vi "Teleop.vi"(10 "Match Info":T1={"Autonomous Elapsed Seconds"=0.0, "TeleOp Elapsed Seconds"=0.0, "Disabled Elapsed Seconds"=0.0, "Visited Autonomous"=FALSE, "Visited TeleOp"=FALSE, "Visited Disabled"=FALSE, "Autonomous Settings"={"Autonomous Style"=enum."Independent", "VI Refnum"=refnum}}, 11 "Call Context":T2) -> ()   [LabVIEW 2020]
doc: "This VI is called for each enabled TeleOp packet received from the DS. It is typically used to read from joysticks and other inputs and update I/O or setpoints for timed control loops. It should complete and return within 20 milliseconds or risk missing DS packets."
uses:
  <vilib>/Rock Robotics/WPI/DriverStation/WPI_DriverStationDerivedRobotMode.ctl
  <vilib>/Rock Robotics/WPI/DriverStation/WPI_DriverStationMatch Info.ctl
  Swerve/Implementation/Swerve Setpoints.ctl
  Swerve/Implementation/Swerve Operations.ctl
  Intake/Implementation/Intake Setpoints.ctl
  Intake/Implementation/Intake Operations.ctl
  <vilib>/Rock Robotics/WPI/Joystick/XBox Buttons Indexer.ctl
  <vilib>/Rock Robotics/WPI/Joystick/XBox Axes Indexer.ctl
  Climber/Implementation/Climber Operations.ctl
  Climber/Implementation/Climber Setpoints.ctl
  Shooter/Implementation/Shooter Operations.ctl
  Shooter/Implementation/Shooter Setpoints.ctl
  <vilib>/Rock Robotics/WPI/Utilities/WPI_GetSetVariantRefNum.vi
  <vilib>/Rock Robotics/Network Tables/NT Write Boolean Array.vi
  <vilib>/Rock Robotics/Network Tables/NT Write Numeric Array.vi
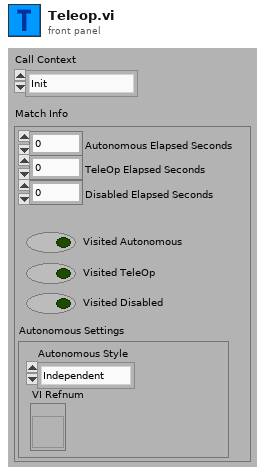
[diagram p1: front panel]
types:
  T1 = typedef "WPI_DriverStationMatch Info.ctl" = cluster{"Autonomous Elapsed Seconds":dbl, "TeleOp Elapsed Seconds":dbl, "Disabled Elapsed Seconds":dbl, "Visited Autonomous":bool, "Visited TeleOp":bool, "Visited Disabled":bool, "Autonomous Settings":cluster{"Autonomous Style":enum16{"Iterative", "Independent"}, "VI Refnum":refnum<vi>}}
  T2 = typedef "WPI_DriverStationDerivedRobotMode.ctl" = enum16{"Init", "Execute", "Stop"}
  T3 = typedef "XBox Buttons Indexer.ctl" = enum16{"A", "B", "X", "Y", "Left Bumper", "Right Bumper", "Back", "Start", "Left Joystick", "Right Joystick"}
  T4 = typedef "XBox Axes Indexer.ctl" = enum16{"Left X", "Left Y", "Left Trigger", "Right Trigger", "Right X", "Right Y"}
  T5 = typedef "Intake Setpoints.ctl" = cluster{"Operation":T6, "Numeric":dbl}
  T6 = typedef "Intake Operations.ctl" = enum16{"Reserve", "Read Current", "Immediate", "Retract", "Extend", "Feed"}
  T7 = typedef "Swerve Setpoints.ctl" = cluster{"Operation":T8, "Gyro":dbl, "X Rotate":dbl, "FWD":dbl, "STR":dbl, "Time":dbl, "Angle":dbl, "Distance":dbl, "Right Trigger":dbl, "Y Rotate":dbl, "Start Angle":dbl}
  T8 = typedef "Swerve Operations.ctl" = enum16{"Reserve", "Read Current", "Immediate", "Direct  Joystick Drive", "Joystick Drive", "Drive for Distance", "Drive for Time", "Turn to Angle", "Drive to Angle(Time)", "Drive to Angle(Distance)"}
  T9 = typedef "WPI_JoystickDevRef.ctl" = cluster{"Device":T10}
  T10 = typedef "WPI_JoystickDeviceEnum.ctl" = enum16{"USB 0", "USB 1", "USB 2", "USB 3", "USB 4", "USB 5"}
  T11 = typedef "Climber Setpoints.ctl" = cluster{"Operation":T12, "Numeric":dbl}
  T12 = typedef "Climber Operations.ctl" = enum16{"Reserve", "Read Current", "Immediate", "Unlock Winch", "Lock Winch", "Stop Winch", "Spool Winch", "Unspool Winch", "Arm Out", "Arm In", "Open Hook", "Close Hook"}
  T13 = typedef "ADIS16470 Device Reference.ctl" = cluster{"DevStatus":errorcluster, "Hardware Config":T14, "Calibration Complete":refnum<notifier>, "Status Reference":refnum<data-value>, "Data Reference":refnum<data-value>, "Sychronous Process VI":T18, "Cmd FIFO":refnum<k33>, "Source":T19, "Data FIFO":refnum<k33>, "Calibration Time (ms)":u32, "Data Reference":refnum<data-value>}
  T14 = typedef "ADIS16470 Hardware Configuration.ctl" = cluster{"SPI Clock Rate (Hz)":dbl, "IMU SPI Mode (3)":T15, "IMU Reset Pin":T16, "IMU SPI Bus":T17, "IMU Data Ready Pin":T16, "Stall Config":cluster{"Pow2BytesPerRead":u8, "StallTicks":u16, "CsToSclkTicks":u8}}
  T15 = typedef "WPI_SPIMode.ctl" = enum16{"Mode 0 (Clk Idle Low,Sample on Leading)", "Mode 1 (Clk Idle Low,Sample on Trailing)", "Mode 2 (Clk Idle High,Sample on Leading)", "Mode 3 (Clk Idle High,Sample on Trailing)"}
  T16 = typedef "FPGA_DIOChannel.ctl" = enum8{"DIO 0", "DIO 1", "DIO 2", "DIO 3", "DIO 4", "DIO 5", "DIO 6", "DIO 7", "DIO 8", "DIO 9", "DIO MXP 0", "DIO MXP 1", "DIO MXP 2", "DIO MXP 3", "DIO MXP 4", "DIO MXP 5", "DIO MXP 6", "DIO MXP 7", "DIO MXP 8", "DIO MXP 9", "DIO MXP 10", "DIO MXP 11", "DIO MXP 12", "DIO MXP 13", "DIO MXP 14", "DIO MXP 15", "SPI Port CS1", "SPI Port CS2", "SPI Port CS3", "SPI Port MISO", "SPI Port MOSI", "Invalid"}
  T17 = typedef "spi_bus.ctl" = enum16{"SPI On-Board, CS0", "SPI On-Board, CS1", "SPI On-Board, CS2", "SPI On-Board, CS3", "SPI MXP", "Invalid"}
  T18 = typedef "ADIS16470 Process.ctl" = refnum<vi>
  T19 = typedef "FPGA_CounterEncoderSourceConvertionLVSourceType.ctl" = cluster{"DevStatus":errorcluster, "AnalogTriggerMode?":bool, "DigitalMode":cluster{"DIO Channel":T20}, "AnalogTriggerMode":cluster{"AnalogTriggerIndex":T21, "OutputType":T22}}
  T20 = typedef "FPGA_DIODigitalSourceChannel.ctl" = enum8{"DIO 0", "DIO 1", "DIO 2", "DIO 3", "DIO 4", "DIO 5", "DIO 6", "DIO 7", "DIO 8", "DIO 9", "DIO MXP 0", "DIO MXP 1", "DIO MXP 2", "DIO MXP 3", "DIO MXP 4", "DIO MXP 5", "DIO MXP 6", "DIO MXP 7", "DIO MXP 8", "DIO MXP 9", "DIO MXP 10", "DIO MXP 11", "DIO MXP 12", "DIO MXP 13", "DIO MXP 14", "DIO MXP 15", "SPI Port CS1", "SPI Port CS2", "SPI Port CS3", "SPI Port MISO", "SPI Port MOSI", "Disabled"}
  T21 = typedef "FPGA_AnalogTriggerIndex.ctl" = enum8{"Trig 0", "Trig 1", "Trig 2", "Trig 3", "Trig 4", "Trig 5", "Trig 6", "Trig 7", "Invalid"}
  T22 = typedef "FPGA_AnalogTriggerOutType.ctl" = enum16{"InWindow", "TriggerState", "Rising", "Falling"}
  T23 = typedef "ADIS16470 Data.ctl" = cluster{"XAngle":dbl, "YAngle":dbl, "ZAngle":dbl}
  T24 = typedef "Shooter Setpoints.ctl" = cluster{"Operation":T25, "Numeric":dbl}
  T25 = typedef "Shooter Operations.ctl" = enum16{"Reserve", "Read Current", "Immediate", "Shoot"}
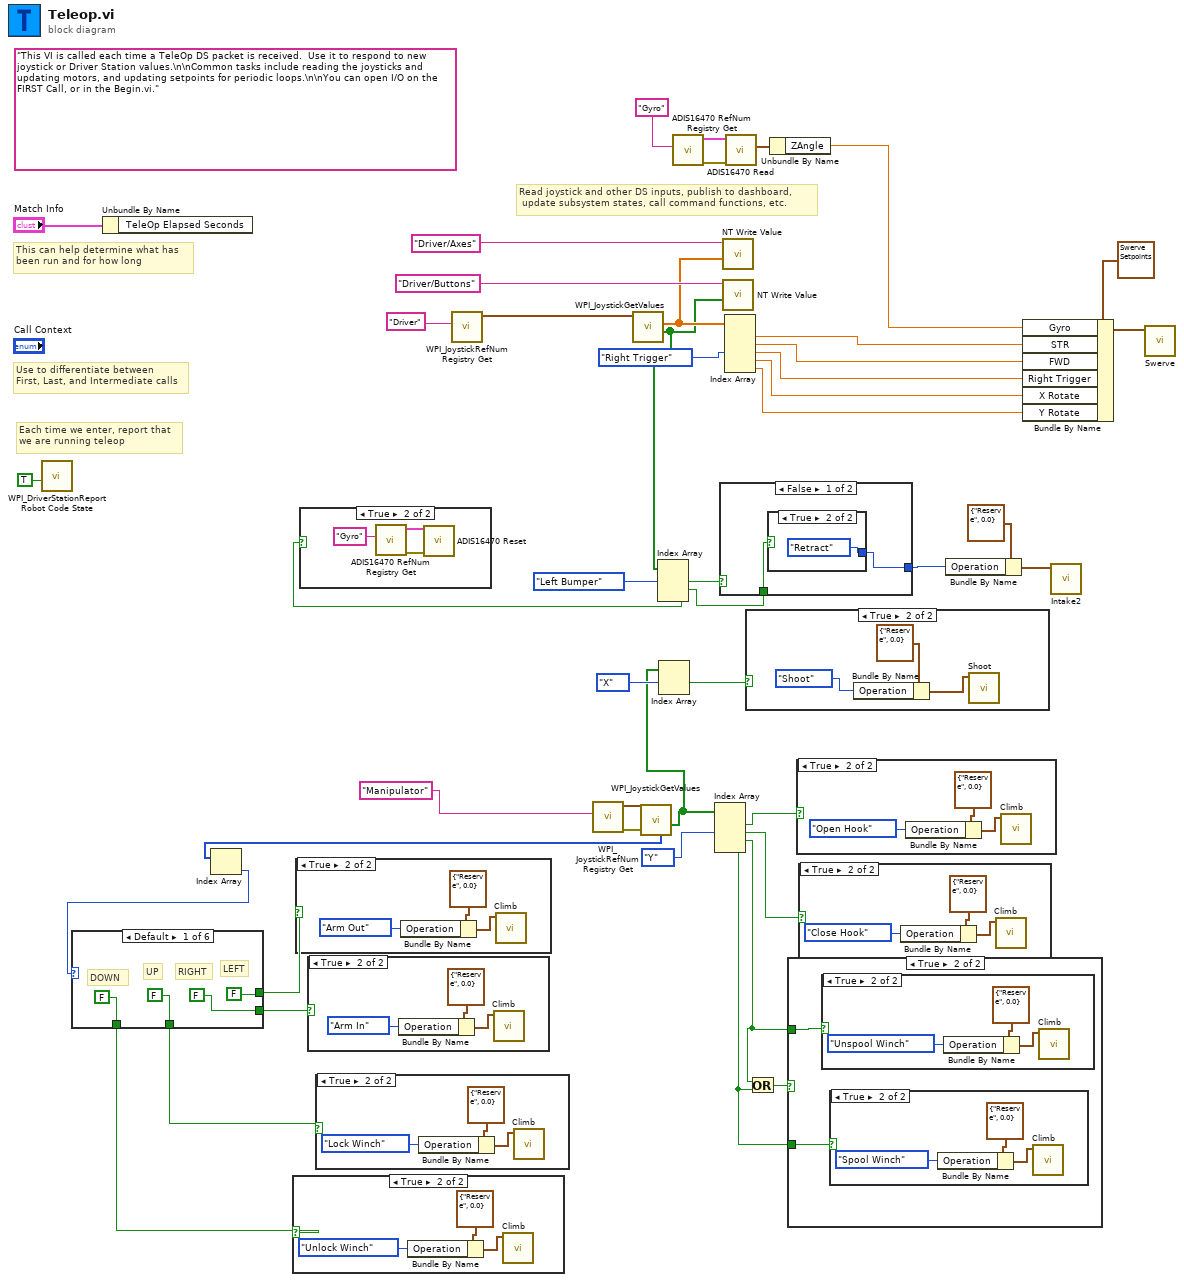
[diagram p0: block diagram]
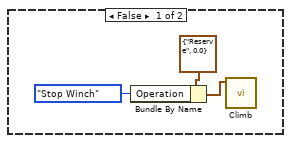
[diagram p2: hidden frame]
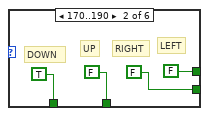
[diagram p11: hidden frame]
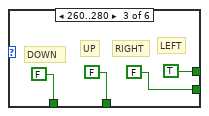
[diagram p12: hidden frame]
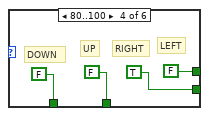
[diagram p13: hidden frame]
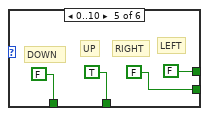
[diagram p14: hidden frame]
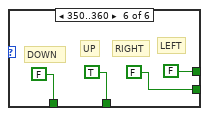
[diagram p15: hidden frame]
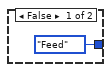
[diagram p18: hidden frame]
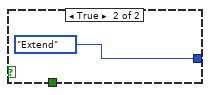
[diagram p19: hidden frame]
diagram:
  (unwired) "This VI is called each time a TeleOp DS packet is received.  Use it to respond to new joystick or Driver Station values.\n\nCommon tasks include reading the joysticks and updating motors, and updating setpoints for periodic loops.\n\nYou can open I/O on the FIRST Call, or in the Begin.vi."
  # "Read joystick and other DS inputs, publish to dashboard,\n update subsystem states, call command functions, etc."
  # "Each time we enter, report that\nwe are running teleop"
  # "Use to differentiate between\nFirst, Last, and Intermediate calls"
  # "This can help determine what has\nbeen run and for how long"
  n1 = call <vilib>:"WPI_DriverStationReport Robot Code State.vi"("TeleOp"=TRUE ("Autonomous")) -> ()  [unwired: 10 in, 1 out]
  n2 = Unbundle By Name("Match Info") -> ()  [unwired: 1 out]
  n3 = call <vilib>:"WPI_JoystickRefNum Registry Get.vi"("refnum name"="Driver") -> ("JoystickDevRef"=w43:T9)  [unwired: 1 in, 9 out]
  n4 = call <vilib>:"WPI_JoystickRefNum Registry Get.vi"("refnum name"="Manipulator") -> ("error out"=w22:errorcluster, "JoystickDevRef"=w23:T9)  [unwired: 1 in, 8 out]
  n5 = call <vilib>:"WPI_JoystickGetValues.vi"("JoystickDevRef"=w43) -> ("Buttons"=w25:bool[], "Axes"=w41:dbl[])  [unwired: 6 in, 3 out]
  n6 = call <vilib>:"WPI_JoystickGetValues.vi"("error in (no error)"=w22, "JoystickDevRef"=w23) -> ("Buttons"=w4:bool[], "POVs"=w20:i16[])  [unwired: 5 in, 3 out]
  n7 = Index Array(array=w20) -> (element=w17:i16)  [unwired: 1 in]
  n8 = case shown="Default" w17 {
    tunnel: [FALSE TRUE FALSE FALSE FALSE FALSE] -> w13
    tunnel: [FALSE FALSE TRUE FALSE FALSE FALSE] -> w15
    tunnel: [FALSE FALSE FALSE TRUE FALSE FALSE] -> w16
    tunnel: [FALSE FALSE FALSE FALSE TRUE TRUE] -> w14
    frame Default {
      # "RIGHT"
      # "LEFT"
      # "UP"
      # "DOWN"
    }
    frame 170..190 {
      # "RIGHT"
      # "LEFT"
      # "UP"
      # "DOWN"
    }
    frame 260..280 {
      # "RIGHT"
      # "LEFT"
      # "UP"
      # "DOWN"
    }
    frame 80..100 {
      # "RIGHT"
      # "LEFT"
      # "UP"
      # "DOWN"
    }
    frame 0..10 {
      # "RIGHT"
      # "LEFT"
      # "UP"
      # "DOWN"
    }
    frame 350..360 {
      # "RIGHT"
      # "LEFT"
      # "UP"
      # "DOWN"
    }
  }
  n9 = case shown="True" w13 {
    frame False {
    }
    frame True {
      n10 = Bundle By Name(cluster=T11 {"Operation"=enum."Reserve", "Numeric"=0.0} ("SubSystem Data"), "Operation"=Climber_Operations."Unlock Winch") -> (w73:T11)
      n11 = call "Climb.vi"("SubSystem Data"=w73) -> ()  [unwired: 10 in, 1 out]
    }
  }
  n12 = case shown="True" w15 {
    frame False {
    }
    frame True {
      n13 = Bundle By Name(cluster=T11 {"Operation"=enum."Reserve", "Numeric"=0.0} ("SubSystem Data"), "Operation"=Climber_Operations."Arm Out") -> (w76:T11)
      n14 = call "Climb.vi"("SubSystem Data"=w76) -> ()  [unwired: 10 in, 1 out]
    }
  }
  n15 = case shown="True" w16 {
    frame False {
    }
    frame True {
      n16 = Bundle By Name(cluster=T11 {"Operation"=enum."Reserve", "Numeric"=0.0} ("SubSystem Data"), "Operation"=Climber_Operations."Arm In") -> (w79:T11)
      n17 = call "Climb.vi"("SubSystem Data"=w79) -> ()  [unwired: 10 in, 1 out]
    }
  }
  n18 = case shown="True" w14 {
    frame False {
    }
    frame True {
      n19 = Bundle By Name(cluster=T11 {"Operation"=enum."Reserve", "Numeric"=0.0} ("SubSystem Data"), "Operation"=Climber_Operations."Lock Winch") -> (w82:T11)
      n20 = call "Climb.vi"("SubSystem Data"=w82) -> ()  [unwired: 10 in, 1 out]
    }
  }
  n21 = Index Array(array=w25, index #1=XBox_Buttons_Indexer."Left Bumper" ("XBox Buttons")) -> (element #1=w28:bool, element #2=w26:bool, element #3=w5:bool)  [unwired: 2 in]
  n22 = case shown="True" w5 {
    frame False {
    }
    frame True {
      n23 = call <vilib>:"ADIS16470 RefNum Registry Get.vi"("refnum name"="Gyro") -> ("error out"=w85:errorcluster, "ADIS16470DevRef out"=w84:T13)  [unwired: 9 in]
      n24 = call <vilib>:"ADIS16470 Reset.vi"("error in (no error)"=w85, "ADIS16470DevRef"=w84) -> ()  [unwired: 8 in, 2 out]
    }
  }
  n25 = Index Array(array=w4, index #1=XBox_Buttons_Indexer."X" ("XBox Buttons")) -> (element #1=w24:bool)  [unwired: 1 in, 1 out]
  n26 = call <vilib>:"ADIS16470 RefNum Registry Get.vi"("refnum name"="Gyro") -> ("error out"=w37:errorcluster, "ADIS16470DevRef out"=w36:T13)  [unwired: 9 in]
  n27 = Index Array(array=w4, index #2=XBox_Buttons_Indexer."Y" ("XBox Buttons")) -> (element #1=w12:bool, element #2=w11:bool, element #3=w1:bool, element #4=w2:bool)  [unwired: 3 in]
  n28 = case shown="False" w28 {
    tunnel: [w87 Intake_Operations."Extend" ("Operation")] -> w27
    tunnel: w26 -> [w86 _]
    frame False {
      n29 = case shown="True" w86 {
        tunnel: [Intake_Operations."Feed" ("Operation") Intake_Operations."Retract" ("Operation")] -> w87
        frame False {
        }
        frame True {
        }
      }
    }
    frame True {
    }
  }
  n30 = call-poly <vilib>:"NT Write Value.vi"("Numeric Array"=w41, "Name"="Driver/Axes") -> ()  [unwired: 9 in, 1 out]
  n31 = call-poly <vilib>:"NT Write Value.vi"("Boolean Array"=w25, "Name"="Driver/Buttons") -> ()  [unwired: 9 in, 1 out]
  n32 = Index Array(array=w41, index #3=XBox_Axes_Indexer."Right Trigger" ("XBox Axes")) -> (element #1=w18:dbl, element #2=w19:dbl, element #3=w32:dbl, element #4=w31:dbl, element #5=w6:dbl)  [unwired: 4 in]
  n33 = call <vilib>:"ADIS16470 Read.vi"("error in (no error)"=w37, "ADIS16470DevRef"=w36) -> ("ADIS16470 Value"=w34:T23)  [unwired: 6 in, 3 out]
  n34 = case shown="True" w24 {
    frame False {
    }
    frame True {
      n35 = Bundle By Name(cluster=T24 {"Operation"=enum."Reserve", "Numeric"=0.0} ("SubSystem Data"), "Operation"=Shooter_Operations."Shoot") -> (w93:T24)
      n36 = call "Shoot.vi"("SubSystem Data"=w93) -> ()  [unwired: 10 in, 1 out]
    }
  }
  n37 = Or(x=w1, y=w2) -> (x .or. y?=w3:bool)
  n38 = Unbundle By Name(w34) -> ("ZAngle"=w33:dbl)
  n39 = case shown="True" w3 {
    tunnel: w1 -> [_ w98]
    tunnel: w2 -> [_ w97]
    frame False {
      n40 = Bundle By Name(cluster=T11 {"Operation"=enum."Reserve", "Numeric"=0.0} ("SubSystem Data"), "Operation"=Climber_Operations."Stop Winch") -> (w96:T11)
      n41 = call "Climb.vi"("SubSystem Data"=w96) -> ()  [unwired: 10 in, 1 out]
    }
    frame True {
      n42 = case shown="True" w98 {
        frame False {
        }
        frame True {
          n43 = Bundle By Name(cluster=T11 {"Operation"=enum."Reserve", "Numeric"=0.0} ("SubSystem Data"), "Operation"=Climber_Operations."Unspool Winch") -> (w104:T11)
          n44 = call "Climb.vi"("SubSystem Data"=w104) -> ()  [unwired: 10 in, 1 out]
        }
      }
      n45 = case shown="True" w97 {
        frame False {
        }
        frame True {
          n46 = Bundle By Name(cluster=T11 {"Operation"=enum."Reserve", "Numeric"=0.0} ("SubSystem Data"), "Operation"=Climber_Operations."Spool Winch") -> (w101:T11)
          n47 = call "Climb.vi"("SubSystem Data"=w101) -> ()  [unwired: 10 in, 1 out]
        }
      }
    }
  }
  n48 = case shown="True" w12 {
    frame False {
    }
    frame True {
      n49 = Bundle By Name(cluster=T11 {"Operation"=enum."Reserve", "Numeric"=0.0} ("SubSystem Data"), "Operation"=Climber_Operations."Open Hook") -> (w107:T11)
      n50 = call "Climb.vi"("SubSystem Data"=w107) -> ()  [unwired: 10 in, 1 out]
    }
  }
  n51 = case shown="True" w11 {
    frame False {
    }
    frame True {
      n52 = Bundle By Name(cluster=T11 {"Operation"=enum."Reserve", "Numeric"=0.0} ("SubSystem Data"), "Operation"=Climber_Operations."Close Hook") -> (w110:T11)
      n53 = call "Climb.vi"("SubSystem Data"=w110) -> ()  [unwired: 10 in, 1 out]
    }
  }
  n54 = Bundle By Name(cluster=T5 {"Operation"=enum."Reserve", "Numeric"=0.0} ("SubSystem Data"), "Operation"=w27) -> (w30:T5)
  n55 = Bundle By Name(cluster=T7 {"Operation"=enum."Joystick Drive", "Gyro"=0.0, "X Rotate"=0.0, "FWD"=0.0, "STR"=0.0, "Time"=0.0, "Angle"=0.0, "Distance"=0.0, "Right Trigger"=0.0, "Y Rotate"=0.0, "Start Angle"=0.0} ("SubSystem Data"), "Gyro"=w33, "STR"=w18, "FWD"=w19, "Right Trigger"=w32, "X Rotate"=w31, "Y Rotate"=w6) -> (w38:T7)
  n56 = call "Intake2.vi"("SubSystem Data"=w30) -> ()  [unwired: 10 in, 1 out]
  n57 = call "Swerve.vi"("SubSystem Data"=w38) -> ()  [unwired: 10 in, 1 out]
